vi "Created Administrator.vi"(8 "error in (no error)":errorcluster, 11 "File Path Control":path) -> (0 "error out":errorcluster, 3 "File Path out":path)   [LabVIEW 2019, in "UserManagement.lvlib" / "UserManagement.lvclass"]
uses:
  UserManagement.lvclass
  User.ctl
  Permission.ctl
  <vilib>/Utility/config.llb/Write Key (String).vi
  <vilib>/Utility/config.llb/NI_LVConfig.lvlib
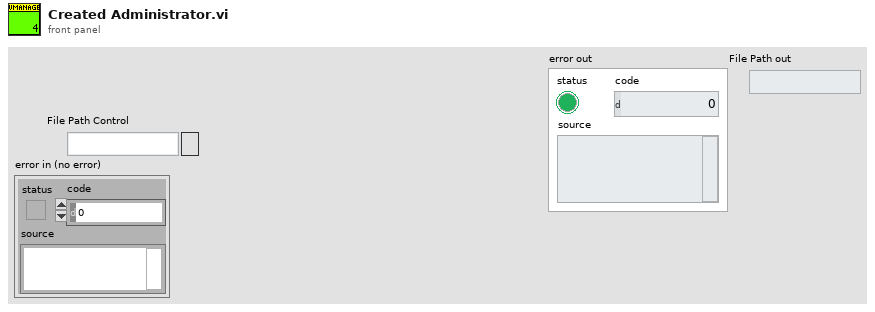
[diagram p1: front panel]
types:
  T1 = typedef "UserManagement.lvlib/UserManagement.lvclass/User.ctl" = cluster{"Permission":T2, "UserName":string, "PassWord":string}
  T2 = typedef "UserManagement.lvlib/UserManagement.lvclass/Permission.ctl" = enum16{"Engineer", "Technical", "Operator"}
  T3 = enum16{"open", "replace", "create", "open or create", "replace or create", "replace or create with confirmation"}
  T4 = typedef "NI_LVConfig.lvlib/Config Data RefNum.ctl" = refnum<k1>
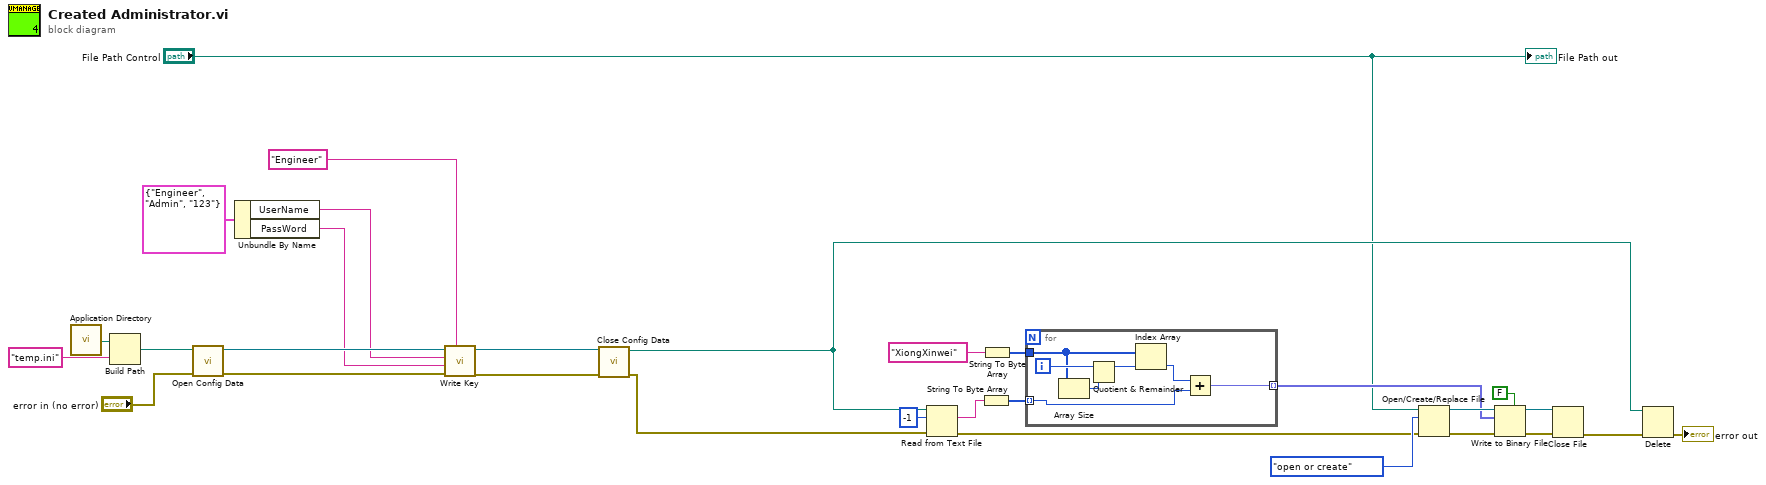
[diagram p0: block diagram]
diagram:
  n1 = call <vilib>:"Application Directory.vi"() -> ("Application Directory"=w30:path)
  n2 = Build Path(base path=w30, name or relative path="temp.ini" ("名称或相对路径")) -> (appended path=w28:path)
  n3 = call <vilib>:"Open Config Data.vi"("error in (no error)"="error in (no error)", "configuration file path"=w28) -> ("error out"=w26:errorcluster, "refnum"=w27:T4)  [unwired: 7 in, 1 out]
  n4 = Unbundle By Name(T1 {"Permission"=enum."Engineer", "UserName"="Admin", "PassWord"="123"} ("input cluster")) -> ("UserName"=w10:string, "PassWord"=w9:string)
  n5 = call-poly <vilib>:"Write Key.vi"("section"="Engineer", "error in (no error)"=w26, "value"=w9, "key"=w10, "refnum"=w27) -> ("error out"=w5:errorcluster, "refnum out"=w6:T4)  [unwired: 4 in, 1 out]
  n6 = call <vilib>:"Close Config Data.vi"("error in (no error)"=w5, "refnum"=w6) -> ("error out"=w13:errorcluster, "file path"=w12:path)  [unwired: 8 in]
  n7 = Read from Text File(file (use dialog)=w12, count=-1 ("计数"), error in=w13) -> (text=w24:string, error out=w1:errorcluster)  [unwired: 1 in, 2 out]
  n8 = String To Byte Array(string=w24) -> (unsigned byte array=w22:u8[])
  n9 = String To Byte Array(string="XiongXinwei" ("字符串")) -> (unsigned byte array=w21:u8[])
  n10 = for {
    tunnel: w22 -> [w33] mode=indexing
    tunnel: w21 -> [w36]
    tunnel: [w32] -> w16 mode=indexing
    i -> [w37]
    n11 = Array Size(array=w36) -> (size(s)=w35:i32)
    n12 = Quotient & Remainder(x=w37, y=w35) -> (x-y*floor(x/y)=w31:i32)  [unwired: 1 out]
    n13 = Index Array(array=w36, index=w31) -> (element=w34:u8)
    n14 = Add ("加")(x=w34, y=w33) -> (x+y=w32:fxp<+,8,8>)
  }
  n15 = Open/Create/Replace File(file path (use dialog)="File Path Control", error in=w1, operation (0:open)=T3."open or create" ("操作(0:open)")) -> (refnum out=w20:refnum<file>, error out=w19:errorcluster)  [unwired: 3 in, 1 out]
  n16 = Write to Binary File(file (use dialog)=w20, data=w16, error in=w19, 5:FALSE ("预置数组或字符串大小？(T)")) -> (refnum out=w18:refnum<file>, error out=w17:errorcluster)  [unwired: 2 in, 1 out]
  n17 = Close File(refnum=w18, error in=w17) -> (error out=w11:errorcluster)  [unwired: 1 out]
  n18 = Delete(path (use dialog)=w12, error in=w11) -> (error out=→"error out":errorcluster)  [unwired: 3 in, 2 out]
  "File Path out" <- "File Path Control"
